vi "Treatment.vi"() -> ()   [LabVIEW 2020]
uses:
  controls/Rename.ctl
  controls/Load.ctl
  controls/CleanSD.ctl
  controls/Save.ctl
  controls/Del.ctl
  controls/Add.ctl
  controls/Average.ctl
  controls/mylistbox.ctl
  controls/SliderSDII.ctl
  controls/Calc.ctl
  controls/AllOffOn.ctl
  controls/Scale_up.ctl
  controls/Norm.ctl
  controls/LeftArrow.ctl
  controls/RightArrow.ctl
  Classes/Control/Control-Client/Control-Client.lvclass
  dependecies/ControlsVIs/Clusters-def/graphs_TR.ctl
  dependecies/ControlsVIs/Clusters-def/Graphs_ref_Client.ctl
  Classes/Control/Control-Client/Control-Client.lvclass/Control-Client.ctl
  Classes/Experiments/Experiments_group.lvclass/Experiments_group.ctl
  dependecies/ControlsVIs/Clusters-def/Types_of_Graphs-Client.ctl
  Classes/Control/Control-Client/methods/Read Group #.vi
  dependecies/globalVarSD.vi
  Classes/Control/Control-Client/Erase color.vi
  Classes/Experiments/Experiments_group.lvclass
panel:
  in  "stop":bool
  in  "VD2_calc_abs":bool
  in  "Right shift kinetics":T1
  in  "Left shift kinetics":T2
  in  "Norm Kinetics":T3
  in  "Scale_up":dbl=1.01 format="%#_3f"
  in  "ScaleUp":T4
  in  "Value":dbl=10.0 format="%#_13g"
  in  "ChangeAll":T5
  in  "NaN Correct":T6
  in  "CalcStability":T7
  out "stability":T8(graph)
  in  "X-scale":bool
  in  "Group title":string
  in  "Del group exp":T9
  in  "Add group":T10
  out "error out":errorcluster
  in  "Exp name":string
  in  "Clean mode":u16(ring)=1 items=["delete", "approx"]
  in  "Clean":T6
  in  "sigma":dbl=1.4 min=0.0 step=0.1
  in  "BG slider":T11={0.0, 16.0} scale=0.0..10.0
  in  "BG correct":T6
  in  "Del exp":T9
  in  "Load Exp":T12
  in  "Save exp":T13
  in  "Save":enum32{"Automatic", "User-def"}(ring)
  in  "Rename exp":T14
  in  "Average exp":T15
  in  "times slider":T11={120.7741935483871, 734.8387096774194} scale=-40.0..74.0 scale format="%#.1f"
  in  "del spec":i32=2 min=2 step=1
  in  "Del spectrum":T9
  in  "Add spectrum":T10
  out "Spectra":cluster{"Y":dbl[], "Y":dbl[]}[](graph)
  in  "waves slider":T11={434.19354838709677, 734.8387096774194} scale=240.824..813.9446 scale format="%#.1f"
  in  "del kin":i32=2 min=2 step=1
  in  "LogY":bool
  in  "Del kinetics":T9
  in  "Add kinetics":T10
  out "Kinetics":cluster{"Y":dbl[], "Y":dbl[]}[](graph)
  in  "folder of the day":string="no title"
  in  "selected wavelengths":dbl[](array[numeric])=[370.0, 400.0, 450.0, 500.0, 550.0, 600.0, 640.0, 700.0]
  out "Exp data graph":dbl[][](graph)
  in  "Commentaires exp":string="...Write experiment description..."
  in  "Experiments":T16=[4]
  in  "Group":u16(ring) items=["1. 17_05_2018-10-30-test"]
  in  "Tab Control":enum32{"Raw data"}(tab)
  in  "correct raw BG":bool
  out "Raw data":cluster{dbl[], dbl[]}[](graph)
  in  "raw bg":i32[](array[numeric])
  out "Raw data BG":cluster{dbl[], dbl[]}[](graph)
  # "copyrights: ELYSE Université Paris-Sud LCP/CNRS UMR8000 Dr. DENISOV Sergey"
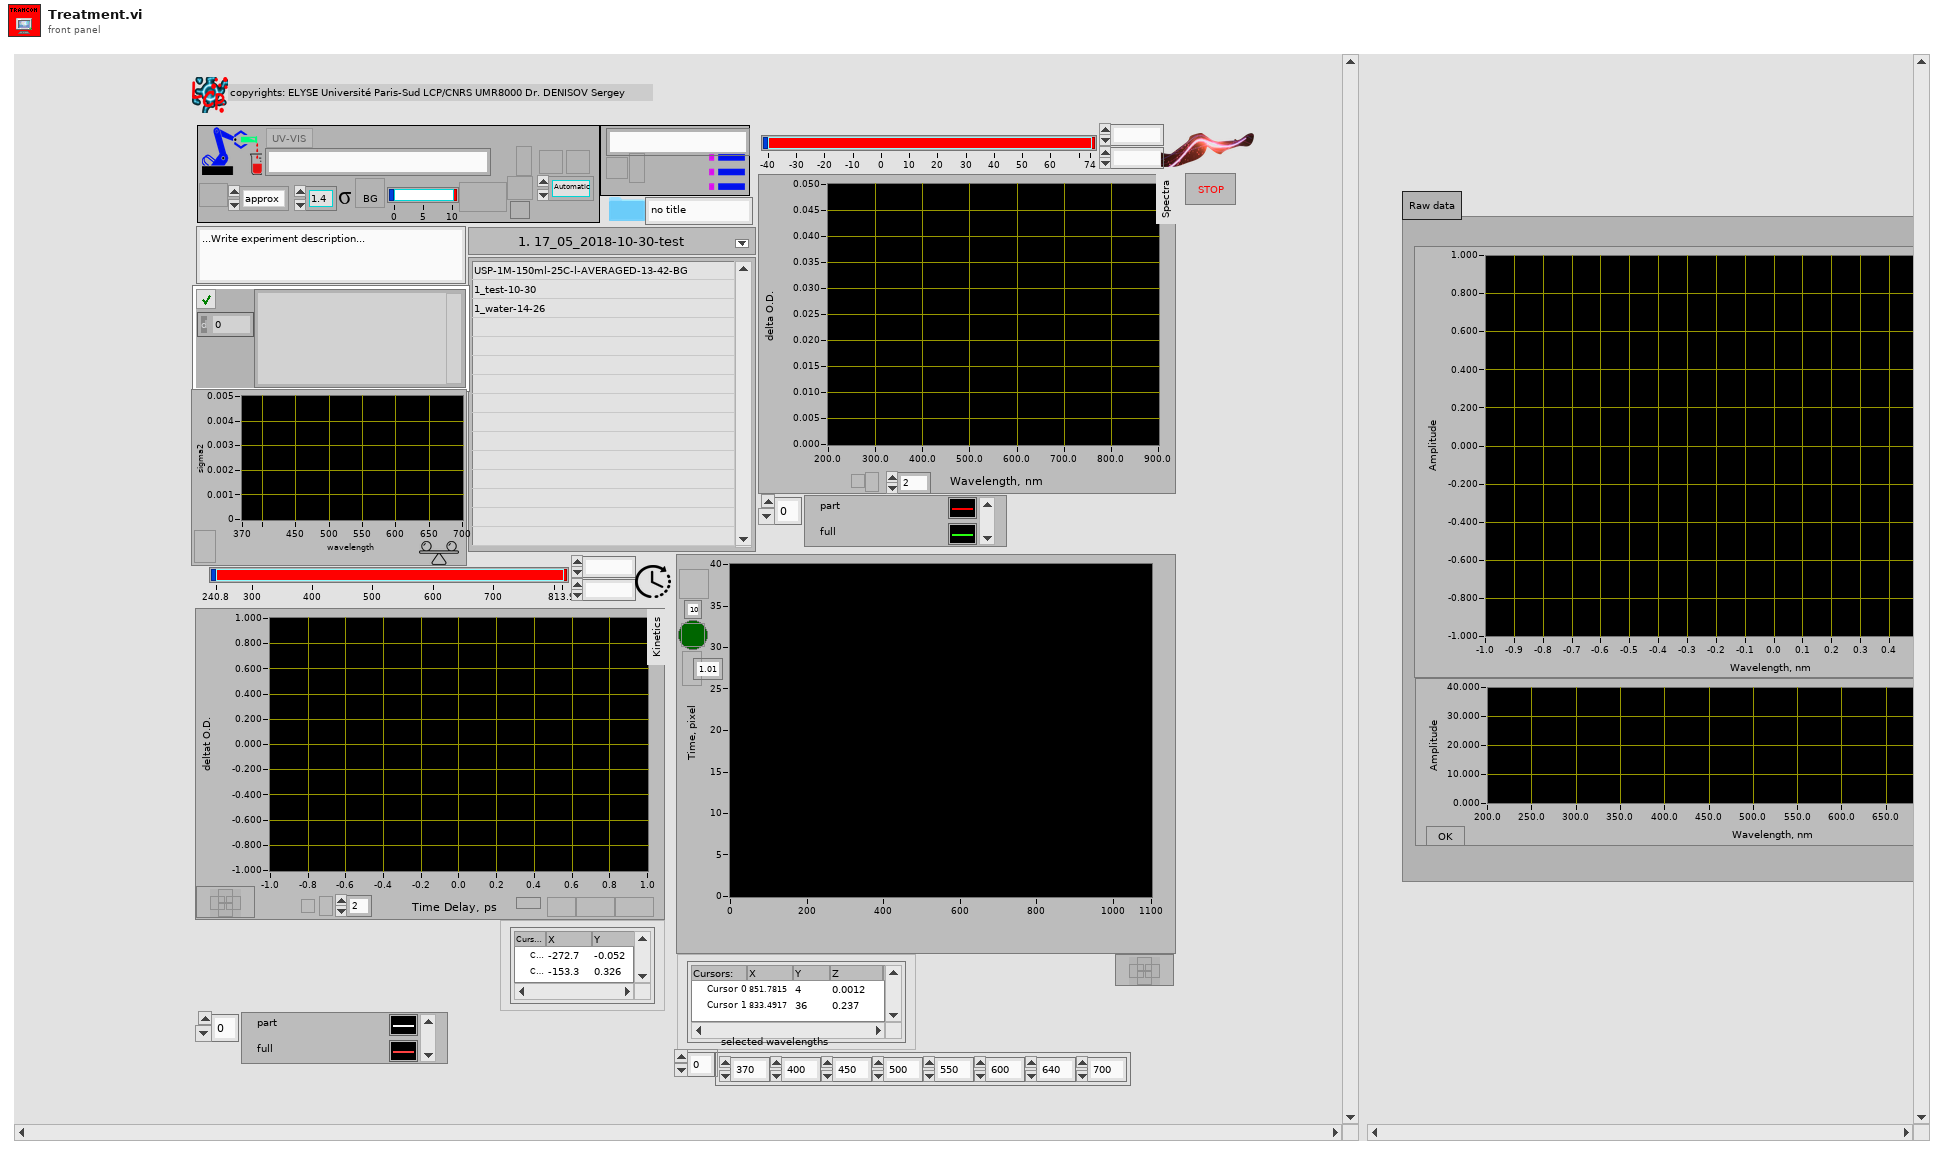
[diagram p1: front panel]
types:
  T1 = typedef "RightArrow.ctl" = bool
  T2 = typedef "LeftArrow.ctl" = bool
  T3 = typedef "Norm.ctl" = bool
  T4 = typedef "Scale_up.ctl" = bool
  T5 = typedef "AllOffOn.ctl" = bool
  T6 = typedef "CleanSD.ctl" = bool
  T7 = typedef "Calc.ctl" = bool
  T8 = cluster{"wavelengths":dbl[], "wavelengths":dbl[]}[]
  T9 = typedef "Del.ctl" = bool
  T10 = typedef "Add.ctl" = bool
  T11 = typedef "SliderSDII.ctl" = cluster{dbl, dbl}
  T12 = typedef "Load.ctl" = bool
  T13 = typedef "Save.ctl" = bool
  T14 = typedef "Rename.ctl" = bool
  T15 = typedef "Average.ctl" = bool
  T16 = typedef "mylistbox.ctl" = i32[]
  T17 = cluster{"waves slider":refnum<vi>, "times slider":refnum<vi>}
  T18 = typedef "Control-Client.lvclass/Graphs_ref_Client.ctl" = cluster{"Exp data graph ref":refnum<vi>, "Kinetics graph ref":refnum<vi>, "Spectrum graph ref":refnum<vi>, "cluster graph TR":T19, "Delays Graph":refnum<vi>, "Oscilloscope":refnum<vi>}
  T19 = typedef "graphs_TR.ctl" = cluster{"TR SC":refnum<vi>, "TR OD":refnum<vi>, "Raw data":refnum<vi>, "Raw data BG":refnum<vi>}
  T20 = cluster{"error out":refnum<vi>, "Experiments":refnum<vi>, "Group":refnum<vi>, "Commentaires exp":refnum<vi>}
  T21 = typedef "Control-Client.lvclass/Types_of_Graphs-Client.ctl" = string
  T22 = cluster{"Value":string, "Value":string, cluster{dbl, dbl, dbl, dbl}}
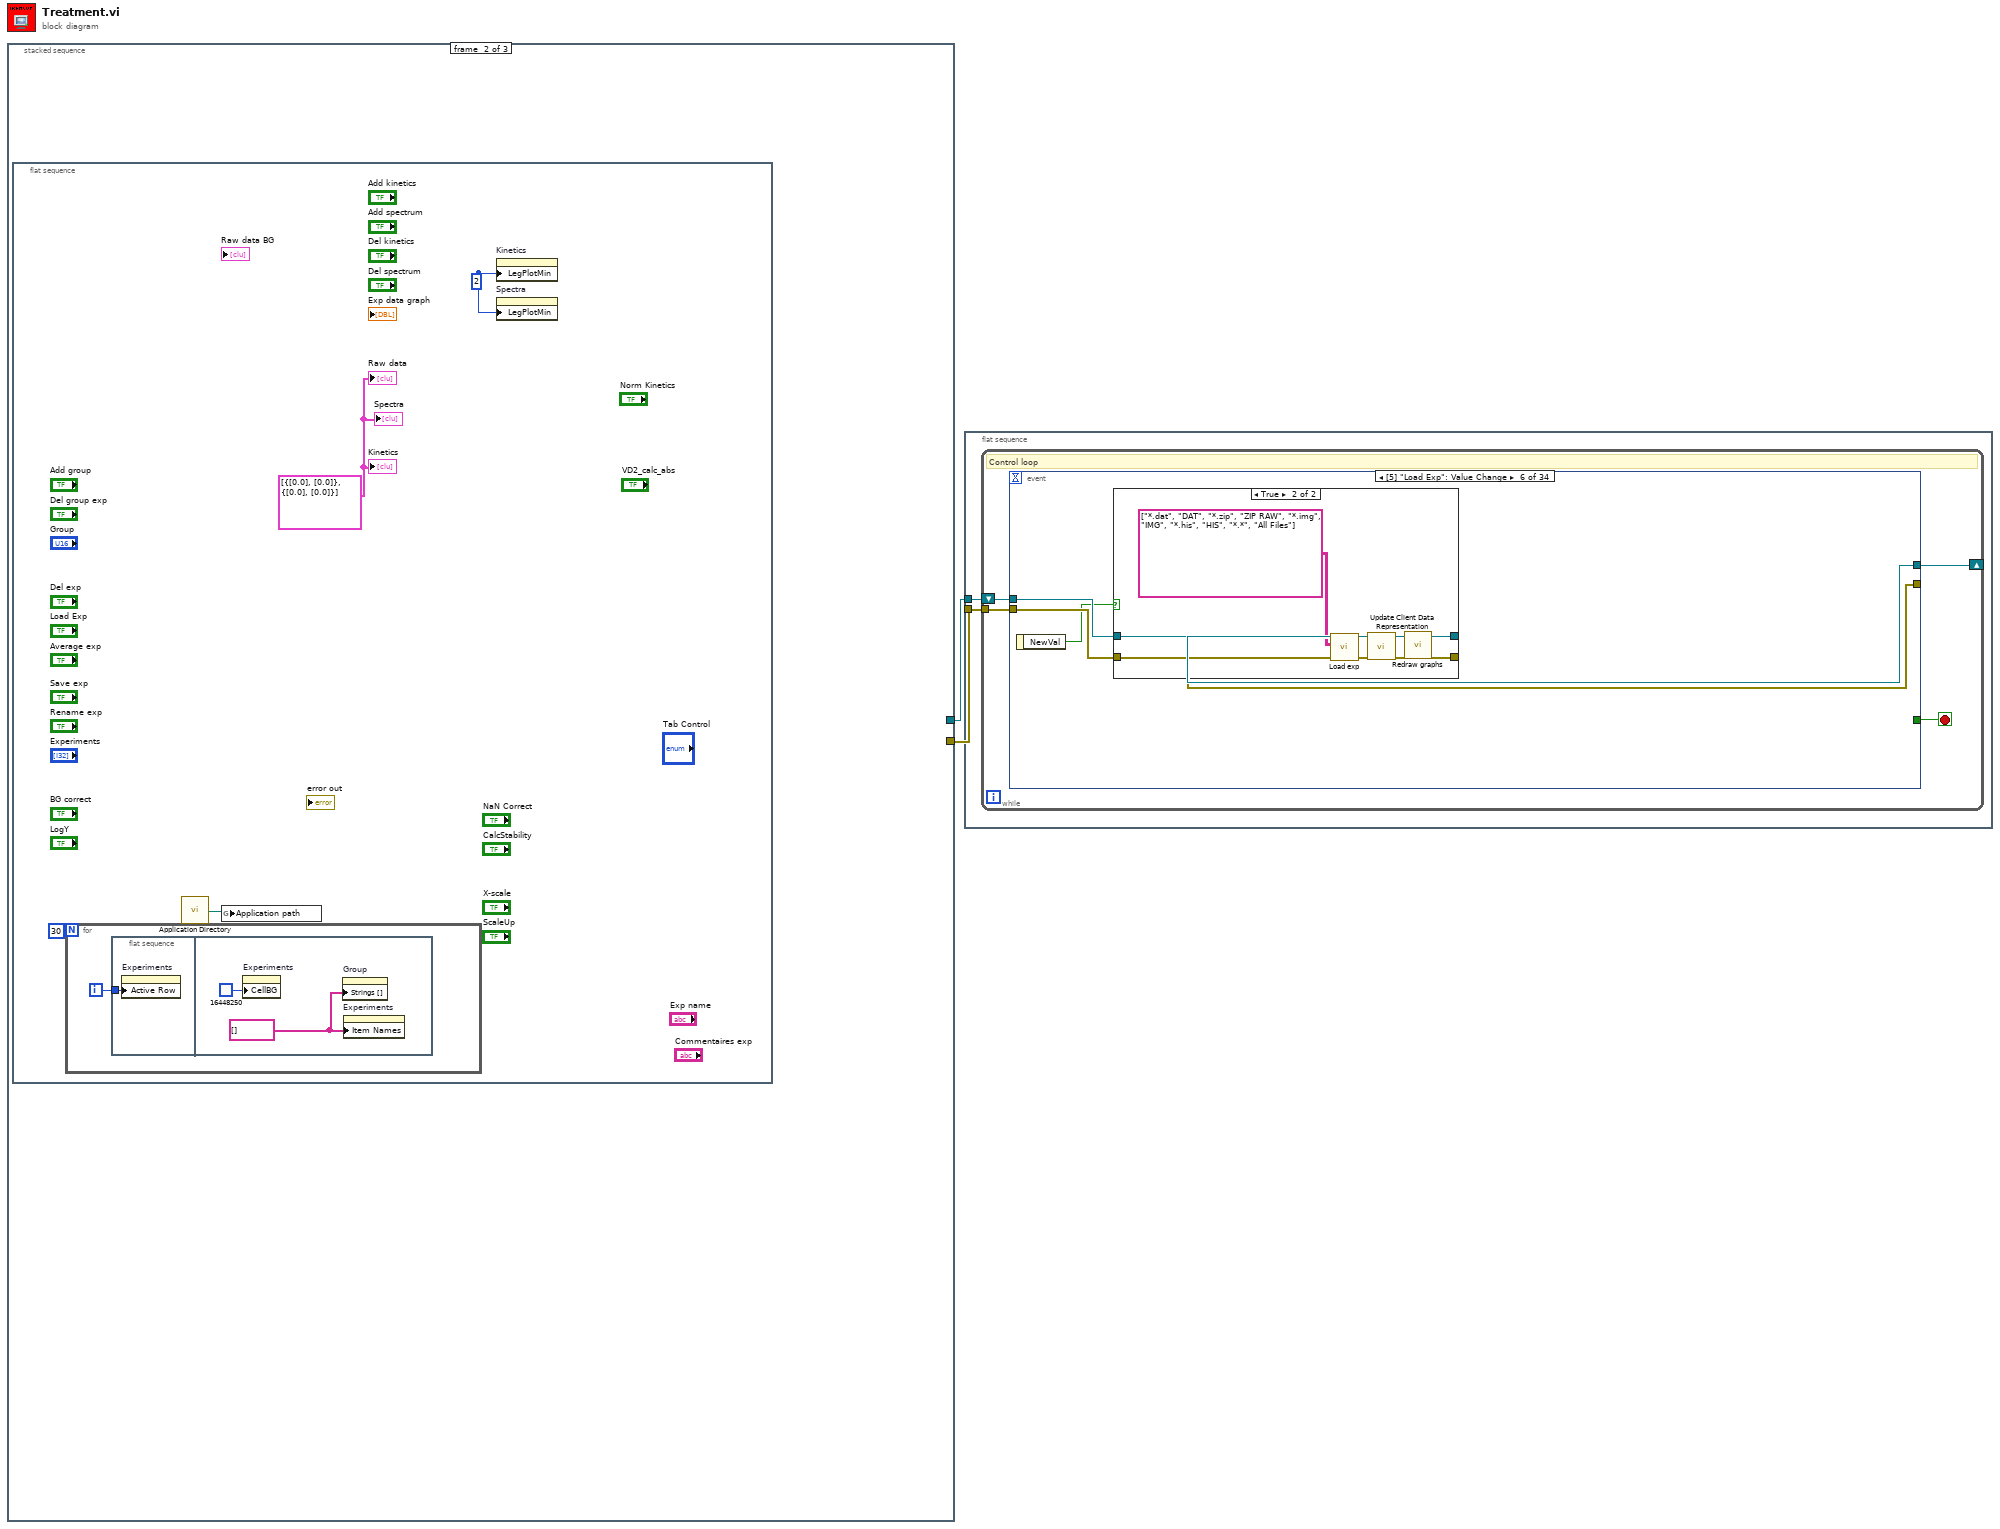
[diagram p0: block diagram]
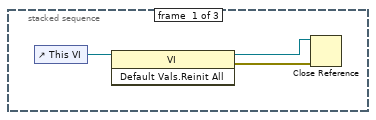
[diagram p2: hidden frame]
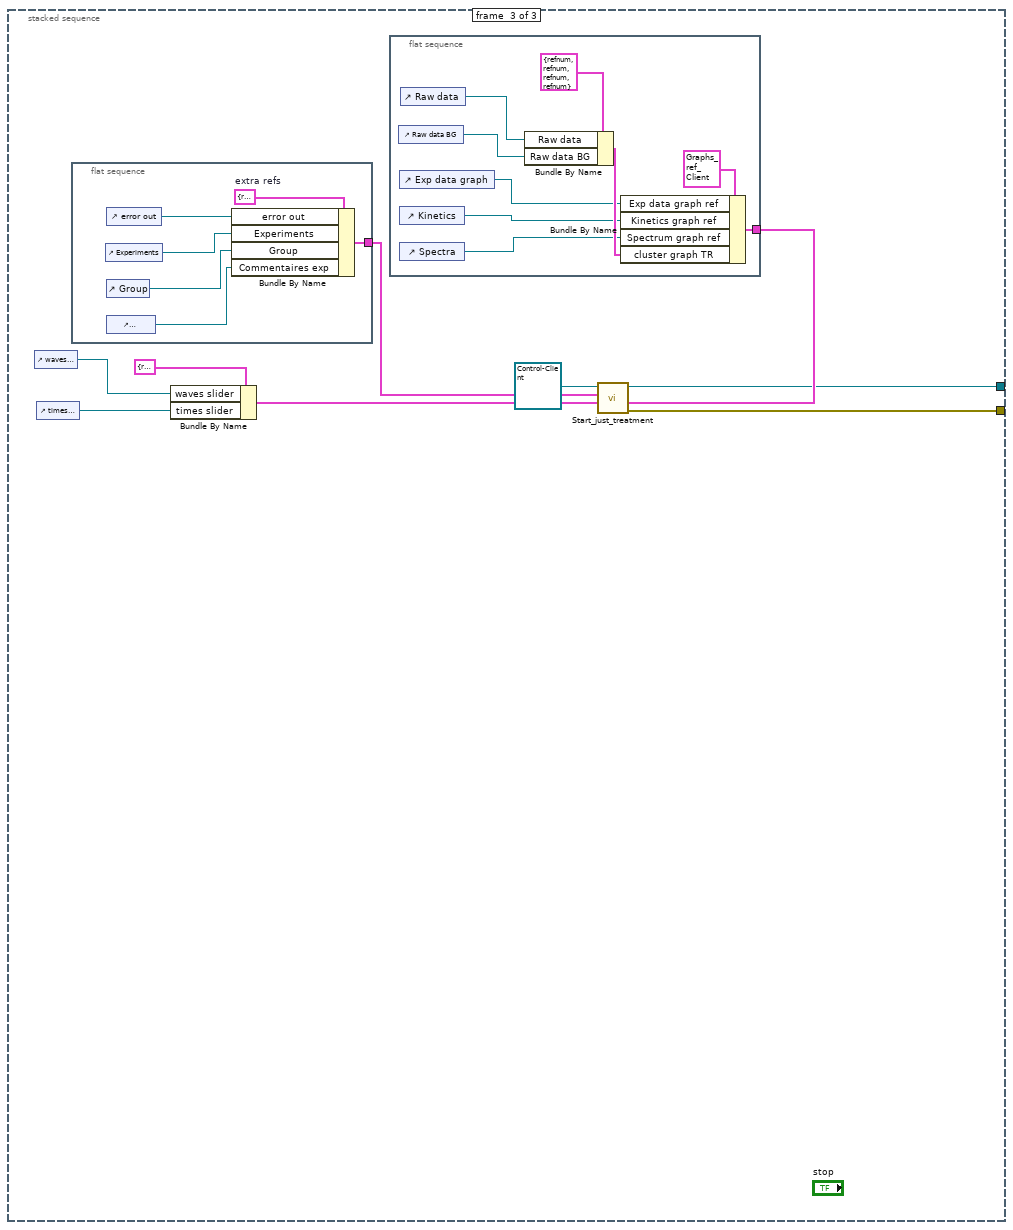
[diagram p3: hidden frame]
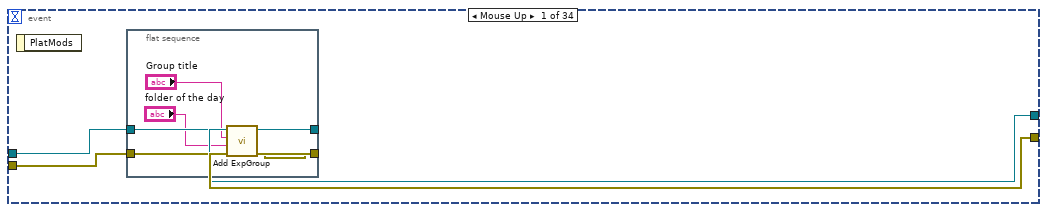
[diagram p4: hidden frame]
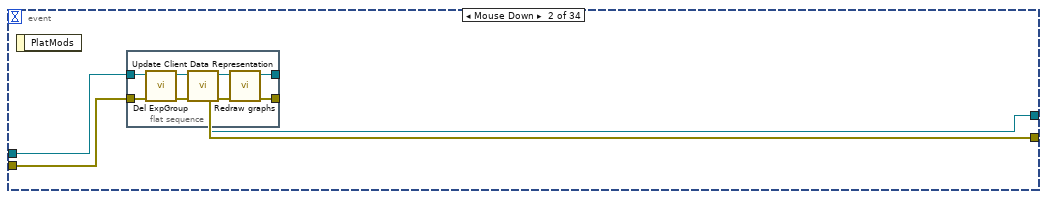
[diagram p5: hidden frame]
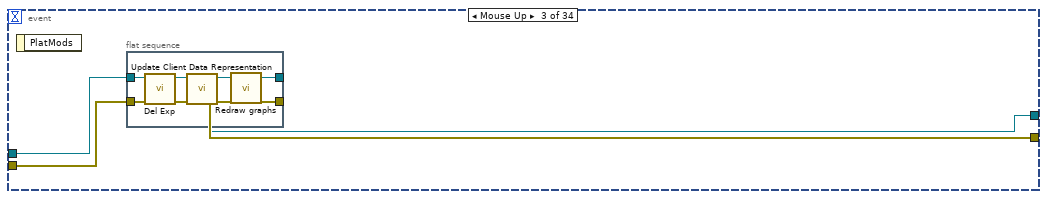
[diagram p6: hidden frame]
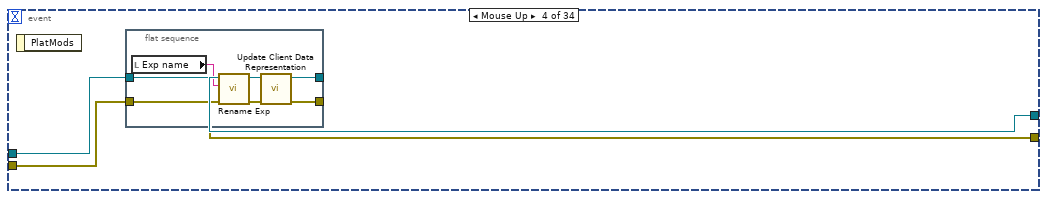
[diagram p7: hidden frame]
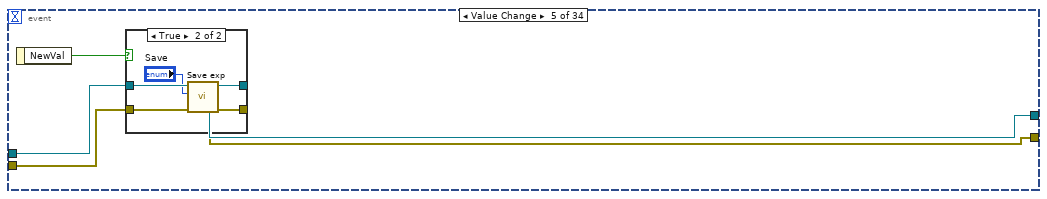
[diagram p8: hidden frame]
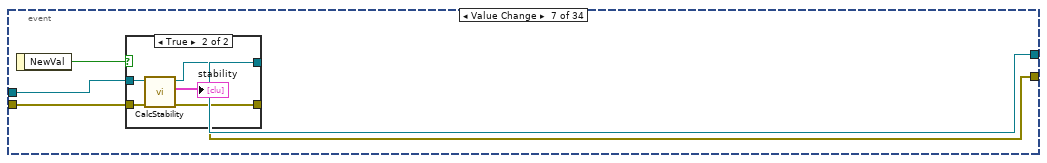
[diagram p11: hidden frame]
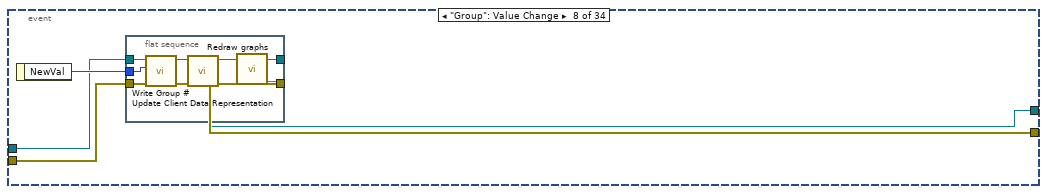
[diagram p13: hidden frame]
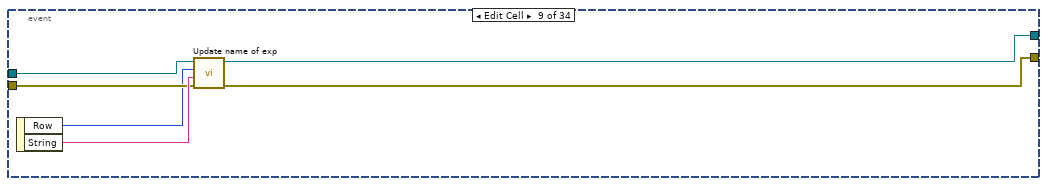
[diagram p14: hidden frame]
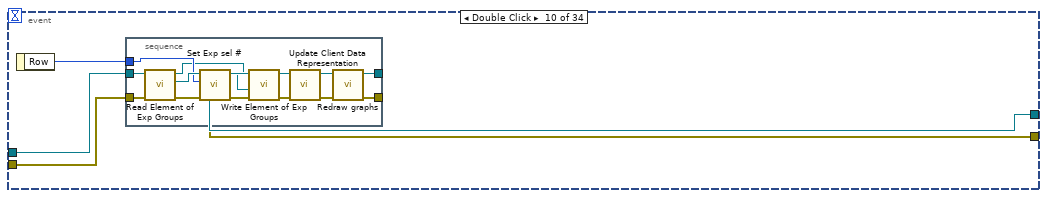
[diagram p15: hidden frame]
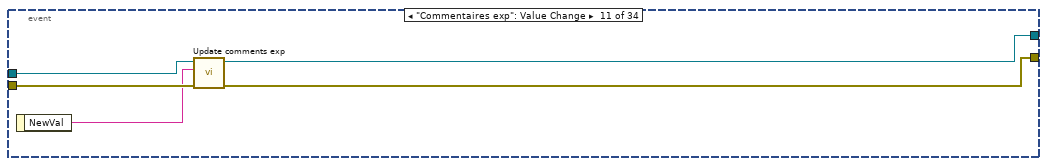
[diagram p16: hidden frame]
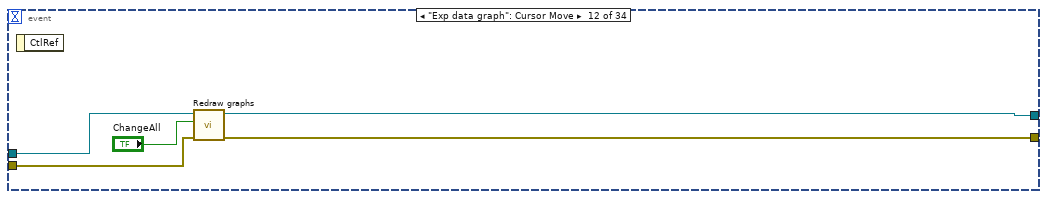
[diagram p17: hidden frame]
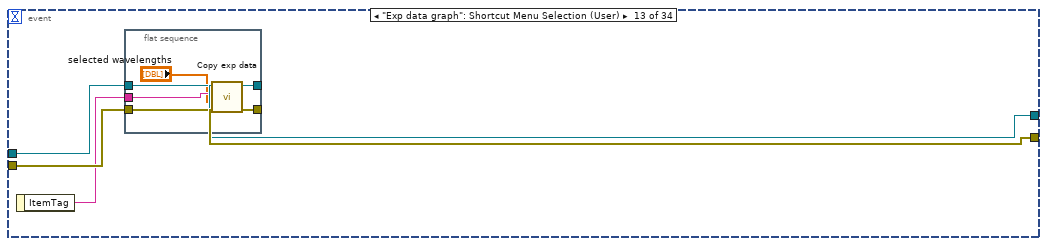
[diagram p18: hidden frame]
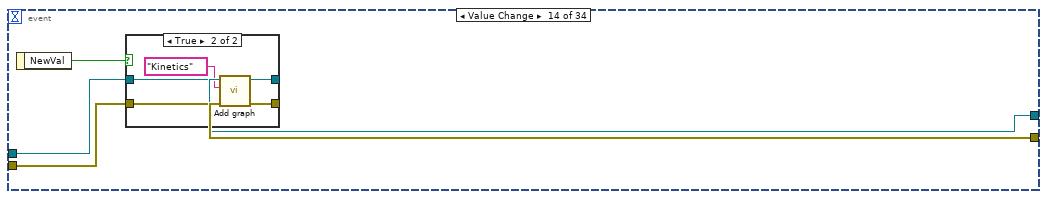
[diagram p19: hidden frame]
diagram:
  n1 = stacked-sequence {
    tunnel: [_ _ w14] -> w2
    tunnel: [_ _ w15] -> w1
    frame #0 {
      n2 = control-ref of="This VI"() -> (w5:refnum<vi>)
      n3 = invoke class="VI" method="Default Vals.Reinit All"(reference=w5) -> (reference out=w4:refnum<vi>, error out=w3:errorcluster)  [unwired: 2 in, 1 out]
      n4 = Close Reference(reference=w4, error in (no error)=w3) -> ()  [unwired: 1 out]
    }
    frame #1 {
      n5 = flat-sequence {
        frame #0 {
          w6 = cluster{dbl[], dbl[]}[] [{[0.0], [0.0]}, {[0.0], [0.0]}] ("Kinetics")
          w7 = u32 2 ("Legend:Plot Minimum")
          n6 = for {
            N: 30 -> [_]
            i -> [w10]
            n7 = flat-sequence {
              tunnel: w10 -> [w11]
              frame #0 {
                n8 = property on="Experiments" class="LstBox (strict)"("Active Row"=w11) -> ()  [unwired: 2 in, 2 out]
              }
              frame #1 {
                w12 = string[] [] ("Item Names")
                n9 = property on="Experiments" class="LstBox (strict)"("CellBG"=u32 16448250) -> ()  [unwired: 2 in, 2 out]
                n10 = property on="Group" class="Ring (strict)"("Strings []"=w12) -> ()  [unwired: 2 in, 2 out]
                n11 = property on="Experiments" class="LstBox (strict)"("Item Names"=w12) -> ()  [unwired: 2 in, 2 out]
              }
            }
          }
          n12 = call <vilib>:"Application Directory.vi"() -> ("Application Directory"=w9:path)
          n13 = global write "globalVarSD.vi" "Application path"(w9) -> ()
          n14 = property on="Kinetics" class="XYGraph (strict)"("LegPlotMin"=w7) -> ()  [unwired: 2 in, 2 out]
          n15 = property on="Spectra" class="XYGraph (strict)"("LegPlotMin"=w7) -> ()  [unwired: 2 in, 2 out]
          "Spectra" <- w6
          "Kinetics" <- w6
          "Raw data" <- w6
        }
      }
    }
    frame #2 {
      n16 = control-ref of="waves slider"() -> (w19:refnum<vi>)
      n17 = control-ref of="times slider"() -> (w20:refnum<vi>)
      n18 = flat-sequence {
        tunnel: [w23] -> w16
        frame #0 {
          w28 = T20 {"error out"=refnum, "Experiments"=refnum, "Group"=refnum, "Commentaires exp"=refnum}  # extra refs
          n19 = control-ref of="Experiments"() -> (w26:refnum<vi>)
          n20 = control-ref of="error out"() -> (w27:refnum<vi>)
          n21 = control-ref of="Group"() -> (w25:refnum<vi>)
          n22 = control-ref of="Commentaires exp"() -> (w24:refnum<vi>)
          n23 = Bundle By Name(cluster=w28, "error out"=w27, "Experiments"=w26, "Group"=w25, "Commentaires exp"=w24) -> (w23:T20)
        }
      }
      n24 = Bundle By Name(cluster=T17 {"waves slider"=refnum, "times slider"=refnum}, "waves slider"=w19, "times slider"=w20) -> (w18:T17)
      n25 = flat-sequence {
        tunnel: [w35] -> w17
        frame #0 {
          n26 = control-ref of="Raw data BG"() -> (w29:refnum<vi>)
          n27 = control-ref of="Exp data graph"() -> (w31:refnum<vi>)
          n28 = control-ref of="Kinetics"() -> (w33:refnum<vi>)
          n29 = control-ref of="Spectra"() -> (w32:refnum<vi>)
          n30 = control-ref of="Raw data"() -> (w30:refnum<vi>)
          n31 = Bundle By Name(cluster=T19 {"TR SC"=refnum, "TR OD"=refnum, "Raw data"=refnum, "Raw data BG"=refnum} ("cluster de sortie"), "Raw data"=w30, "Raw data BG"=w29) -> (w34:T19)
          n32 = Bundle By Name(cluster=T18 {"Exp data graph ref"=refnum, "Kinetics graph ref"=refnum, "Spectrum graph ref"=refnum, "cluster graph TR"={"TR SC"=refnum, "TR OD"=refnum, "Raw data"=refnum, "Raw data BG"=refnum}, "Delays Graph"=refnum, "Oscilloscope"=refnum} ("Graph refs"), "Exp data graph ref"=w31, "Kinetics graph ref"=w33, "Spectrum graph ref"=w32, "cluster graph TR"=w34) -> (w35:T18)
        }
      }
      n33 = call "Start_just_treatment.vi"("Graph refs"=w17, "Slider cluster"=w18, "extra refs"=w16, "Control-Client in"=refnum<class "Control-Client.lvclass"> refnum) -> ("error out"=w14:errorcluster, "Control-Client out"=w15:refnum<class "Control-Client.lvclass">)  [unwired: 6 in]
    }
  }
  n34 = flat-sequence {
    tunnel: w2 -> [w39]
    tunnel: w1 -> [w38]
    frame #0 {
      n35 = while "Control Loop" {
        tunnel: w39 -> [w43]
        shift-right: [w41] -> _
        shift-left: w38 -> [w42]
        stop <- w40 stop-if-true
        # "Control loop"
        n36 = event shown="[5] \"Load Exp\": Value Change" {
          selector: _ -> [_ _ _ _ _ _ _ _ _ _ _ _ _ _ _ _ _ _ _ _ _ _ _ _ _ _ _ _ _ _ _ _ _ _]
          dyn-events: _ -> [_ _ _ _ _ _ _ _ _ _ _ _ _ _ _ _ _ _ _ _ _ _ _ _ _ _ _ _ _ _ _ _ _ _]
          timeout: _ -> [_ _ _ _ _ _ _ _ _ _ _ _ _ _ _ _ _ _ _ _ _ _ _ _ _ _ _ _ _ _ _ _ _ _]
          tunnel: w43 -> [w47 w57 w67 w80 w89 w104 w117 w129 w146 w152 w171 w176 w181 w191 w203 w213 w230 w263 w276 w288 w298 w301 w307 w317 w341 w371 w383 w412 w428 w439 w447 w460 w494 w504]
          tunnel: [w46 w55 w69 w78 w90 w102 w118 w132 w145 w149 w170 w173 w180 w190 w202 w214 w226 w261 w274 w287 w298 w301 w306 w316 w339 w372 w384 w413 w427 w439 w445 w459 w495 w504] -> _
          tunnel: w42 -> [w45 w56 w66 w81 w92 w105 w120 w130 w147 w151 w172 w177 w182 w192 w204 w216 w228 w264 w277 w289 w299 w302 w308 w318 w342 w374 w386 w415 w429 w440 w448 w461 w492 w505]
          tunnel: [w44 w54 w68 w79 w91 w103 w119 w131 w144 w150 w169 w175 w178 w189 w201 w215 w227 w262 w275 w290 w299 w302 w305 w315 w340 w373 w385 w414 w426 w440 w446 w462 w493 w505] -> w41
          tunnel: [_ _ _ _ _ _ _ _ _ _ _ _ _ _ _ _ _ _ _ _ _ _ _ _ _ _ _ _ _ _ _ _ _ w503] -> w40
          event Mouse Up {
            n37 = event-data() -> ()  [unwired: 1 in, 1 out]
            n38 = flat-sequence {
              tunnel: w47 -> [w53]
              tunnel: [w49] -> w46
              tunnel: w45 -> [w52]
              tunnel: [w50] -> w44
              frame #0 {
                n39 = call "Add ExpGroup.vi"("error in (no error)"=w53, "folder of the day"="folder of the day", "Group title"="Group title", "Control-Client in"=w52) -> ("error out"=w49:errorcluster, "Control-Client out"=w50:refnum<class "Control-Client.lvclass">)  [unwired: 6 in]
              }
            }
          }
          event Mouse Down {
            n40 = event-data() -> ()  [unwired: 1 in, 1 out]
            n41 = flat-sequence {
              tunnel: w57 -> [w65]
              tunnel: w56 -> [w64]
              tunnel: [w63] -> w55
              tunnel: [w62] -> w54
              frame #0 {
                n42 = call "Del ExpGroup.vi"("error in (no error)"=w65, "Control-Client in"=w64) -> ("error out"=w58:errorcluster, "Control-Client out"=w59:refnum<class "Control-Client.lvclass">)  [unwired: 8 in]
                n43 = call "Update Client Data Representation.vi"("error in (no error)"=w58, "Control-Client in"=w59) -> ("error out"=w61:errorcluster, "Control-Client out"=w60:refnum<class "Control-Client.lvclass">)  [unwired: 8 in]
                n44 = call "Redraw graphs.vi"("error in (no error)"=w61, "Control-Client in"=w60) -> ("error out"=w63:errorcluster, "Control-Client out"=w62:refnum<class "Control-Client.lvclass">)  [unwired: 8 in]
              }
            }
          }
          event Mouse Up {
            n45 = event-data() -> ()  [unwired: 1 in, 1 out]
            n46 = flat-sequence {
              tunnel: [w77] -> w69
              tunnel: [w76] -> w68
              tunnel: w67 -> [w75]
              tunnel: w66 -> [w74]
              frame #0 {
                n47 = call "Del Exp.vi"("error in (no error)"=w75, "Control-Client in"=w74) -> ("error out"=w72:errorcluster, "Control-Client out"=w73:refnum<class "Control-Client.lvclass">)  [unwired: 8 in]
                n48 = call "Update Client Data Representation.vi"("error in (no error)"=w72, "Control-Client in"=w73) -> ("error out"=w71:errorcluster, "Control-Client out"=w70:refnum<class "Control-Client.lvclass">)  [unwired: 8 in]
                n49 = call "Redraw graphs.vi"("error in (no error)"=w71, "Control-Client in"=w70) -> ("error out"=w77:errorcluster, "Control-Client out"=w76:refnum<class "Control-Client.lvclass">)  [unwired: 8 in]
              }
            }
          }
          event Mouse Up {
            n50 = event-data() -> ()  [unwired: 1 in, 1 out]
            n51 = flat-sequence {
              tunnel: w81 -> [w88]
              tunnel: w80 -> [w87]
              tunnel: [w86] -> w79
              tunnel: [w85] -> w78
              frame #0 {
                n52 = local read "Exp name"() -> (w84:string)
                n53 = call "Rename Exp.vi"("error in (no error)"=w87, "New exp name"=w84, "Control-Client in"=w88) -> ("error out"=w82:errorcluster, "Control-Client out"=w83:refnum<class "Control-Client.lvclass">)  [unwired: 7 in]
                n54 = call "Update Client Data Representation.vi"("error in (no error)"=w82, "Control-Client in"=w83) -> ("error out"=w85:errorcluster, "Control-Client out"=w86:refnum<class "Control-Client.lvclass">)  [unwired: 8 in]
              }
            }
          }
          event Value Change {
            n55 = event-data() -> ("NewVal"=w93:T13)  [unwired: 1 in]
            n56 = case shown="True" w93 {
              tunnel: w92 -> [w95 w100]
              tunnel: [w95 w99] -> w91
              tunnel: [w94 w96] -> w90
              tunnel: w89 -> [w94 w98]
              frame False {
              }
              frame True {
                n57 = call "Save exp.vi"("error in (no error)"=w98, "save"="Save", "Control-Client in"=w100) -> ("error out"=w96:errorcluster, "Control-Client out"=w99:refnum<class "Control-Client.lvclass">)  [unwired: 7 in]
              }
            }
          }
          event Value Change {
            n58 = event-data() -> ("NewVal"=w101:T12)  [unwired: 1 in]
            n59 = case shown="True" w101 {
              tunnel: w105 -> [w107 w116]
              tunnel: w104 -> [w106 w115]
              tunnel: [w107 w109] -> w103
              tunnel: [w106 w110] -> w102
              frame False {
              }
              frame True {
                n60 = call "Load exp.vi"("error in (no error)"=w115, "Files of Type"=string[][] [["*.dat", "DAT"], ["*.zip", "ZIP RAW"], ["*.img", "IMG"], ["*.his", "HIS"], ["*.*", "All Files"]], "Control-Client in"=w116) -> ("error out"=w112:errorcluster, "Control-Client out"=w113:refnum<class "Control-Client.lvclass">)  [unwired: 7 in]
                n61 = call "Update Client Data Representation.vi"("error in (no error)"=w112, "Control-Client in"=w113) -> ("error out"=w111:errorcluster, "Control-Client out"=w114:refnum<class "Control-Client.lvclass">)  [unwired: 8 in]
                n62 = call "Redraw graphs.vi"("error in (no error)"=w111, "Control-Client in"=w114) -> ("error out"=w110:errorcluster, "Control-Client out"=w109:refnum<class "Control-Client.lvclass">)  [unwired: 8 in]
              }
            }
          }
          event Value Change {
            n63 = event-data() -> ("NewVal"=w121:T7)  [unwired: 1 in]
            n64 = case shown="True" w121 {
              tunnel: [w123 w126] -> w119
              tunnel: w120 -> [w123 w125]
              tunnel: [w122 w127] -> w118
              tunnel: w117 -> [w122 w128]
              frame False {
              }
              frame True {
                n65 = call "CalcStability.vi"("error in (no error)"=w128, "Control-Client in"=w125) -> ("error out"=w127:errorcluster, "stability"=→"stability":T8, "Control-Client out"=w126:refnum<class "Control-Client.lvclass">)  [unwired: 7 in]
              }
            }
          }
          event "Group": Value Change {
            n66 = event-data() -> ("NewVal"=w133:u16)  [unwired: 1 in]
            n67 = flat-sequence {
              tunnel: w133 -> [w138]
              tunnel: [w134] -> w132
              tunnel: [w135] -> w131
              tunnel: w130 -> [w140]
              tunnel: w129 -> [w139]
              frame #0 {
                n68 = call "Write Group #.vi"("error in (no error)"=w139, "Group #"=w138, "Control-Client in"=w140) -> ("error out"=w142:errorcluster, "Control-Client out"=w141:refnum<class "Control-Client.lvclass">)  [unwired: 7 in]
                n69 = call "Update Client Data Representation.vi"("error in (no error)"=w142, "Control-Client in"=w141) -> ("error out"=w137:errorcluster, "Control-Client out"=w136:refnum<class "Control-Client.lvclass">)  [unwired: 8 in]
                n70 = call "Redraw graphs.vi"("error in (no error)"=w137, "Control-Client in"=w136) -> ("error out"=w134:errorcluster, "Control-Client out"=w135:refnum<class "Control-Client.lvclass">)  [unwired: 8 in]
              }
            }
          }
          event Edit Cell {
            n71 = event-data() -> ("Row"=w143:i32, "String"=w148:string)  [unwired: 1 in]
            n72 = call "Update name of exp.vi"("error in (no error)"=w146, "Exp name"=w148, "Exp #"=w143, "Control-Client in"=w147) -> ("error out"=w145:errorcluster, "Control-Client out"=w144:refnum<class "Control-Client.lvclass">)  [unwired: 6 in]
          }
          event Double Click {
            n73 = event-data() -> ("Row"=w153:i32)  [unwired: 1 in]
            n74 = stacked-sequence {
              tunnel: w153 -> [w166]
              tunnel: w152 -> [w164]
              tunnel: w151 -> [w163]
              tunnel: [w154] -> w150
              tunnel: [w155] -> w149
              frame #0 {
                n75 = call "Read Element of Exp Groups.vi"("error in (no error)"=w164, "Control-Client in"=w163) -> ("error out"=w165:errorcluster, "Experiments_group.lvclass"=w167:refnum<class "Experiments_group.lvclass">, "Control-Client out"=w161:refnum<class "Control-Client.lvclass">)  [unwired: 7 in]
                n76 = call "Set Exp sel #.vi"("error in (no error)"=w165, "Exp sel #"=w166, "Experiments_group in"=w167) -> ("error out"=w160:errorcluster, "Experiments_group out"=w162:refnum<class "Experiments_group.lvclass">)  [unwired: 7 in]
                n77 = call "Write Element of Exp Groups.vi"("error in (no error)"=w160, "Experiments_group.lvclass"=w162, "Control-Client in"=w161) -> ("error out"=w159:errorcluster, "Control-Client out"=w158:refnum<class "Control-Client.lvclass">)  [unwired: 7 in]
                n78 = call "Update Client Data Representation.vi"("error in (no error)"=w159, "Control-Client in"=w158) -> ("error out"=w156:errorcluster, "Control-Client out"=w157:refnum<class "Control-Client.lvclass">)  [unwired: 8 in]
                n79 = call "Redraw graphs.vi"("error in (no error)"=w156, "Control-Client in"=w157) -> ("error out"=w155:errorcluster, "Control-Client out"=w154:refnum<class "Control-Client.lvclass">)  [unwired: 8 in]
              }
            }
          }
          event "Commentaires exp": Value Change {
            n80 = event-data() -> ("NewVal"=w168:string)  [unwired: 1 in]
            n81 = call "Update comments exp.vi"("error in (no error)"=w171, "Commentaires"=w168, "Control-Client in"=w172) -> ("error out"=w170:errorcluster, "Control-Client out"=w169:refnum<class "Control-Client.lvclass">)  [unwired: 7 in]
          }
          event "Exp data graph": Cursor Move {
            n82 = event-data() -> ()  [unwired: 1 in, 1 out]
            n83 = call "Redraw graphs.vi"("error in (no error)"=w176, "ChangeAll"="ChangeAll", "Control-Client in"=w177) -> ("error out"=w173:errorcluster, "Control-Client out"=w175:refnum<class "Control-Client.lvclass">)  [unwired: 7 in]
          }
          event "Exp data graph": Shortcut Menu Selection (User) {
            n84 = event-data() -> ("ItemTag"=w179:string)  [unwired: 1 in]
            n85 = flat-sequence {
              tunnel: w182 -> [w188]
              tunnel: w181 -> [w187]
              tunnel: [w186] -> w180
              tunnel: [w185] -> w178
              tunnel: w179 -> [w184]
              frame #0 {
                n86 = call "Copy exp data.vi"("error in (no error)"=w187, "selected wavelengths"="selected wavelengths", "ItemTag"=w184, "Control-Client in"=w188) -> ("error out"=w186:errorcluster, "Control-Client out"=w185:refnum<class "Control-Client.lvclass">)  [unwired: 6 in]
              }
            }
          }
          event Value Change {
            n87 = event-data() -> ("NewVal"=w193:T10)  [unwired: 1 in]
            n88 = case shown="True" w193 {
              tunnel: w192 -> [w195 w200]
              tunnel: w191 -> [w194 w199]
              tunnel: [w194 w198] -> w190
              tunnel: [w195 w197] -> w189
              frame False {
              }
              frame True {
                n89 = call "Add graph.vi"("error in (no error)"=w199, "Combo Box"="Kinetics", "Control-Client in"=w200) -> ("error out"=w198:errorcluster, "Control-Client out"=w197:refnum<class "Control-Client.lvclass">)  [unwired: 7 in]
              }
            }
          }
          event Value Change {
            n90 = event-data() -> ("NewVal"=w205:T10)  [unwired: 1 in]
            n91 = case shown="True" w205 {
              tunnel: w204 -> [w207 w212]
              tunnel: w203 -> [w206 w211]
              tunnel: [w206 w210] -> w202
              tunnel: [w207 w209] -> w201
              frame False {
              }
              frame True {
                n92 = call "Add graph.vi"("error in (no error)"=w211, "Combo Box"="Spectra", "Control-Client in"=w212) -> ("error out"=w210:errorcluster, "Control-Client out"=w209:refnum<class "Control-Client.lvclass">)  [unwired: 7 in]
              }
            }
          }
          event Value Change {
            n93 = event-data() -> ("NewVal"=w217:T3)  [unwired: 1 in, 5 out]
            n94 = case shown="True" w217 {
              tunnel: w216 -> [w219 w225]
              tunnel: [w219 w224] -> w215
              tunnel: [w218 w223] -> w214
              tunnel: w213 -> [w218 w222]
              frame False {
              }
              frame True {
                n95 = local read "del kin"() -> (w220:i32)
                n96 = call "Norm graph.vi"("error in (no error)"=w222, "#kinetics"=w220, "Combo Box"="Kinetics", "Control-Client in"=w225) -> ("error out"=w223:errorcluster, "Control-Client out"=w224:refnum<class "Control-Client.lvclass">)  [unwired: 6 in]
              }
            }
          }
          event Value Change {
            n97 = event-data() -> ("CtlRef"=w231:refnum<vi>, "NewVal"=w229:variant)  [unwired: 1 in]
            n98 = flat-sequence {
              tunnel: w231 -> [w241]
              tunnel: w230 -> [w240]
              tunnel: w229 -> [w239]
              tunnel: w228 -> [w236]
              tunnel: [w235] -> w227
              tunnel: [w234] -> w226
              frame #0 {
                n99 = property class="Bool (strict)"(reference=w241, error in=w240) -> (error out=w238:errorcluster, "ClassName"=w232:string)  [unwired: 1 out]
                n100 = case shown="\"Boolean\"" w232 {
                  tunnel: [TRUE w256] -> w237
                  tunnel: [w254 w259] -> w233
                  tunnel: w239 -> [_ w258]
                  tunnel: w238 -> [w254 w257]
                  frame "Digital", Default {
                    (unwired) FALSE
                  }
                  frame "Boolean" {
                    n101 = Variant To Data(error in=w257, type=TRUE, Variant=w258) -> (data=w256:bool, error out=w259:errorcluster)
                  }
                }
                n102 = case shown="True" w237 {
                  tunnel: w236 -> [w243 w251]
                  tunnel: [w243 w250] -> w235
                  tunnel: [w242 w249] -> w234
                  tunnel: w233 -> [w242 w248]
                  frame False {
                  }
                  frame True {
                    n103 = case shown="False" "Left shift kinetics" {
                      tunnel: [0.5 -0.5] -> w244
                      frame False {
                      }
                      frame True {
                      }
                    }
                    n104 = local read "del kin"() -> (w247:i32)
                    n105 = call "Shift X kinetics.vi"("shift"=w244, "error in (no error)"=w248, "#kinetics"=w247, "Combo Box"="Kinetics", "Control-Client in"=w251) -> ("error out"=w249:errorcluster, "Control-Client out"=w250:refnum<class "Control-Client.lvclass">)  [unwired: 5 in]
                  }
                }
              }
            }
          }
          event Value Change {
            n106 = event-data() -> ("NewVal"=w265:T9)  [unwired: 1 in]
            n107 = case shown="True" w265 {
              tunnel: w264 -> [w267 w273]
              tunnel: w263 -> [w266 w272]
              tunnel: [w267 w270] -> w262
              tunnel: [w266 w269] -> w261
              frame False {
              }
              frame True {
                n108 = call "Del graph.vi"("error in (no error)"=w272, "selected graph"="del kin", "Combo Box"="Kinetics", "Control-Client in"=w273) -> ("error out"=w269:errorcluster, "Control-Client out"=w270:refnum<class "Control-Client.lvclass">)  [unwired: 6 in]
              }
            }
          }
          event Value Change {
            n109 = event-data() -> ("NewVal"=w278:T9)  [unwired: 1 in]
            n110 = case shown="True" w278 {
              tunnel: w277 -> [w280 w286]
              tunnel: w276 -> [w279 w285]
              tunnel: [w280 w283] -> w275
              tunnel: [w279 w282] -> w274
              frame False {
              }
              frame True {
                n111 = call "Del graph.vi"("error in (no error)"=w285, "selected graph"="del spec", "Combo Box"="Spectra", "Control-Client in"=w286) -> ("error out"=w282:errorcluster, "Control-Client out"=w283:refnum<class "Control-Client.lvclass">)  [unwired: 6 in]
              }
            }
          }
          event "Kinetics": Shortcut Menu Selection (User) {
            n112 = event-data() -> ("ItemTag"=w291:string)  [unwired: 1 in]
            n113 = flat-sequence {
              tunnel: w291 -> [w297]
              tunnel: [w295] -> w290
              tunnel: w289 -> [w294]
              tunnel: w288 -> [w293]
              tunnel: [w292] -> w287
              frame #0 {
                n114 = call "Copy from XY graph.vi"("error in (no error)"=w293, "ItemTag"=w297, "Type of graph"="Kinetics" ("Combo Box"), "Control-Client in"=w294) -> ("error out"=w292:errorcluster, "Control-Client out"=w295:refnum<class "Control-Client.lvclass">)  [unwired: 6 in]
              }
            }
          }
          event "Spectra": Plot Attribute Change {
            n115 = event-data() -> ("PlotIdx"=w300:i32)  [unwired: 1 in]
            n116 = property on="Spectra" class="XYGraph (strict)"("Active Plot"=w300) -> ()  [unwired: 2 in, 2 out]
          }
          event "Kinetics": Plot Attribute Change {
            n117 = event-data() -> ("PlotIdx"=w303:i32)  [unwired: 1 in]
            n118 = property on="Kinetics" class="XYGraph (strict)"("Active Plot"=w303) -> ()  [unwired: 2 in, 2 out]
          }
          event "Spectra": Shortcut Menu Selection (User) {
            n119 = event-data() -> ("ItemTag"=w304:string)  [unwired: 1 in]
            n120 = flat-sequence {
              tunnel: w308 -> [w314]
              tunnel: w307 -> [w313]
              tunnel: [w312] -> w306
              tunnel: [w311] -> w305
              tunnel: w304 -> [w310]
              frame #0 {
                n121 = call "Copy from XY graph.vi"("error in (no error)"=w313, "ItemTag"=w310, "Type of graph"=T21 "Spectra" ("Combo Box"), "Control-Client in"=w314) -> ("error out"=w312:errorcluster, "Control-Client out"=w311:refnum<class "Control-Client.lvclass">)  [unwired: 6 in]
              }
            }
          }
          event Value Change {
            n122 = event-data() -> ("NewVal"=w319:T15)  [unwired: 1 in]
            n123 = case shown="True" w319 {
              tunnel: [w321 w335] -> w315
              tunnel: w318 -> [w321 w336]
              tunnel: w317 -> [w320 w333]
              tunnel: [w320 w334] -> w316
              frame False {
              }
              frame True {
                n124 = local read "waves slider"() -> (w329:T11)
                n125 = local read "times slider"() -> (w326:T11)
                n126 = property on="Commentaires exp" class="Str"() -> ("Value"=w332:string)  [unwired: 2 in, 2 out]
                n127 = property on="Exp name" class="Str"() -> ("Value"=w331:string)  [unwired: 2 in, 2 out]
                n128 = Unbundle(w326) -> (w325:dbl, w324:dbl)
                n129 = Unbundle(w329) -> (w328:dbl, w327:dbl)
                n130 = Bundle "bounds"(w325, w324, w328, w327) -> (w323:cluster{dbl, dbl, dbl, dbl})  [unwired: 1 in]
                n131 = Bundle("Value"=w331, "Value"=w332, w323) -> (w322:T22)  [unwired: 1 in]
                n132 = call "Average experiments.vi"("error in (no error)"=w333, "sigma"="sigma", "Name+Comments+bounds"=w322, "Control-Client in"=w336) -> ("error out"=w334:errorcluster, "Control-Client out"=w335:refnum<class "Control-Client.lvclass">)  [unwired: 6 in]
              }
            }
          }
          event Value Change {
            n133 = event-data() -> ("CtlRef"=w338:refnum<vi>, "NewVal"=w337:variant)  [unwired: 1 in]
            n134 = flat-sequence {
              tunnel: w342 -> [w352]
              tunnel: w341 -> [w344]
              tunnel: [w348] -> w340
              tunnel: [w347] -> w339
              tunnel: w338 -> [w351]
              tunnel: w337 -> [w346]
              frame #0 {
                n135 = property class="Ctl"(reference=w351) -> ("ClassName"=w350:string)  [unwired: 1 in, 2 out]
                n136 = case shown="\"Boolean\"" w350 {
                  tunnel: [FALSE w369] -> w349
                  tunnel: w346 -> [_ w370]
                  tunnel: [TRUE w368] -> w345
                  tunnel: w344 -> [w363 w367]
                  tunnel: [w363 w366] -> w343
                  frame "Digital", Default {
                  }
                  frame "Boolean" {
                    w369 = TRUE
                    n137 = Variant To Data(error in=w367, type=w369, Variant=w370) -> (data=w368:bool, error out=w366:errorcluster)
                  }
                }
                n138 = case shown="True" w345 {
                  tunnel: w352 -> [w354 w362]
                  tunnel: w343 -> [w353 w361]
                  tunnel: w349 -> [_ w360]
                  tunnel: [w354 w359] -> w348
                  tunnel: [w353 w358] -> w347
                  frame False {
                  }
                  frame True {
                    n139 = Unbundle("BG slider") -> (w355:dbl, w356:dbl)
                    n140 = call "BG correction.vi"("Change?"=w360, "error in (no error)"=w361, "def pixel upper"=w356, "def pixel lower"=w355, "Control-Client in"=w362) -> ("error out"=w358:errorcluster, "Control-Client out"=w359:refnum<class "Control-Client.lvclass">)  [unwired: 5 in]
                  }
                }
              }
            }
          }
          event "correct raw BG": Value Change {
            n141 = event-data() -> ("NewVal"=w375:bool)  [unwired: 1 in, 2 out]
            n142 = case shown="True" w375 {
              tunnel: w374 -> [w377 w382]
              tunnel: [w377 w381] -> w373
              tunnel: [w376 w380] -> w372
              tunnel: w371 -> [w376 w379]
              frame False {
              }
              frame True {
                n143 = call "Raw_BG_correction.vi"("error in (no error)"=w379, "raw bg"="raw bg", "Control-Client in"=w382) -> ("error out"=w380:errorcluster, "Control-Client out"=w381:refnum<class "Control-Client.lvclass">)  [unwired: 7 in]
              }
            }
          }
          event Value Change; "Kinetics": Cursor Move {
            n144 = event-data() -> ("CtlRef"=w387:refnum<vi>)  [unwired: 1 in]
            n145 = flat-sequence {
              tunnel: w387 -> [w393]
              tunnel: w386 -> [w392]
              tunnel: [w391] -> w385
              tunnel: [w390] -> w384
              tunnel: w383 -> [w389]
              frame #0 {
                n146 = property class="Ctl"(reference=w393, error in=w389) -> (error out=w388:errorcluster, "ClassName"=w397:string)  [unwired: 1 out]
                n147 = case shown="\"XYGraph\", Default" w397 {
                  tunnel: [FALSE TRUE] -> w396
                  tunnel: [TRUE "Clean"] -> w395
                  tunnel: [w406 w409] -> w394
                  tunnel: w388 -> [w406 w409]
                  frame "XYGraph", Default {
                  }
                  frame "Boolean" {
                  }
                }
                n148 = case shown="True" w395 {
                  tunnel: w394 -> [w399 w404]
                  tunnel: w396 -> [_ w403]
                  tunnel: [w399 w400] -> w390
                  tunnel: w392 -> [w398 w405]
                  tunnel: [w398 w401] -> w391
                  frame False {
                  }
                  frame True {
                    n149 = call "CursorKinGraphMove.vi"("error in (no error)"=w404, "change"=w403, "Clean mode"="Clean mode", "Control-Client in"=w405) -> ("error out"=w400:errorcluster, "Control-Client out"=w401:refnum<class "Control-Client.lvclass">)  [unwired: 6 in]
                  }
                }
              }
            }
          }
          event Value Change {
            n150 = event-data() -> ()  [unwired: 1 in, 1 out]
            n151 = flat-sequence {
              tunnel: w415 -> [w424]
              tunnel: [w423] -> w414
              tunnel: [w422] -> w413
              tunnel: w412 -> [w421]
              frame #0 {
                n152 = local read "ChangeAll"() -> (w416:T5)
                n153 = Unbundle("waves slider") -> (w418:dbl, w417:dbl)
                n154 = call "Change FromToWave_or_Time.vi"("ChangeAll"=w416, "Combo Box"=T21 "Spectra", "error in (no error)"=w421, "To"=w417, "From"=w418, "Control-Client in"=w424) -> ("error out"=w422:errorcluster, "Control-Client out"=w423:refnum<class "Control-Client.lvclass">)  [unwired: 4 in]
              }
            }
          }
          event Value Change {
            n155 = event-data() -> ("NewVal"=w425:T11)  [unwired: 1 in]
            n156 = flat-sequence {
              tunnel: w429 -> [w438]
              tunnel: [w437] -> w426
              tunnel: [w436] -> w427
              tunnel: w428 -> [w435]
              tunnel: w425 -> [_]
              frame #0 {
                n157 = local read "ChangeAll"() -> (w430:T5)
                n158 = Unbundle("times slider") -> (w431:dbl, w432:dbl)
                n159 = call "Change FromToWave_or_Time.vi"("ChangeAll"=w430, "Combo Box"=T21 "Kinetics", "error in (no error)"=w435, "To"=w432, "From"=w431, "Control-Client in"=w438) -> ("error out"=w436:errorcluster, "Control-Client out"=w437:refnum<class "Control-Client.lvclass">)  [unwired: 4 in]
              }
            }
          }
          event "LogY": Value Change {
            n160 = event-data() -> ("NewVal"=w441:bool)  [unwired: 1 in]
            n161 = flat-sequence {
              tunnel: w441 -> [w443]
              frame #0 {
                n162 = Boolean To (0,1)(Boolean=w443) -> (0, 1=w442:i16)
                n163 = property on="Kinetics" class="XYGraph (strict)"("YScale.Mapping Mode"=w442) -> ()  [unwired: 2 in, 2 out]
              }
            }
          }
          event Value Change {
            n164 = event-data() -> ("NewVal"=w444:T6)  [unwired: 1 in]
            n165 = case shown="True" w444 {
              tunnel: w448 -> [w450 w456]
              tunnel: w447 -> [w449 w455]
              tunnel: [w450 w453] -> w446
              tunnel: [w449 w454] -> w445
              frame False {
              }
              frame True {
                n166 = local read "ChangeAll"() -> (w452:T5)
                n167 = call "NaNCorrect.vi"("error in (no error)"=w455, "Value"="Value", "CorrectAll"=w452, "Control-Client in"=w456) -> ("error out"=w454:errorcluster, "Control-Client out"=w453:refnum<class "Control-Client.lvclass">)  [unwired: 6 in]
              }
            }
          }
          event "Scale_up": Value Change {
            n168 = event-data() -> ("CtlRef"=w458:refnum<vi>, "NewVal"=w457:variant)  [unwired: 1 in]
            n169 = flat-sequence {
              tunnel: [w474] -> w462
              tunnel: w461 -> [w473]
              tunnel: w460 -> [w472]
              tunnel: [w471] -> w459
              tunnel: w458 -> [w470]
              tunnel: w457 -> [w469]
              frame #0 {
                n170 = property class="Ctl"(reference=w470, error in=w472) -> (error out=w463:errorcluster, "ClassName"=w468:string)  [unwired: 1 out]
                n171 = case shown="\"Boolean\"" w468 {
                  tunnel: [FALSE w490] -> w465
                  tunnel: [TRUE w486] -> w464
                  tunnel: [w483 w489] -> w466
                  tunnel: w469 -> [_ w488]
                  tunnel: w463 -> [w483 w487]
                  frame "Digital", Default {
                  }
                  frame "Boolean" {
                    w490 = TRUE
                    n172 = Variant To Data(error in=w487, type=w490, Variant=w488) -> (data=w486:bool, error out=w489:errorcluster)
                  }
                }
                n173 = case shown="True" w464 {
                  tunnel: w473 -> [w476 w482]
                  tunnel: w466 -> [w475 w481]
                  tunnel: [w475 w480] -> w471
                  tunnel: [w476 w479] -> w474
                  tunnel: "Scale_up" -> [_ w478]
                  tunnel: w465 -> [_ w477]
                  frame False {
                  }
                  frame True {
                    n174 = call "ScaleUp correction.vi"("error in (no error)"=w481, "Change?"=w477, "ScaleUp"=w478, "Control-Client in"=w482) -> ("error out"=w480:errorcluster, "Control-Client out"=w479:refnum<class "Control-Client.lvclass">)  [unwired: 6 in]
                  }
                }
              }
            }
          }
          event "VD2_calc_abs": Value Change {
            n175 = event-data() -> ("NewVal"=w491:bool)  [unwired: 1 in, 5 out]
            n176 = case shown="True" w491 {
              tunnel: [w497 w501] -> w495
              tunnel: w494 -> [w497 w502]
              tunnel: [w496 w499] -> w493
              tunnel: w492 -> [w496 w500]
              frame False {
              }
              frame True {
                n177 = property on="Exp name" class="Str"() -> ("Value"=w498:string)  [unwired: 2 in, 2 out]
                n178 = call "VD2_TRABS_Calc.vi"("error in (no error)"=w502, "Exp name"=w498, "Control-Client in"=w500) -> ("error out"=w501:errorcluster, "Control-Client out"=w499:refnum<class "Control-Client.lvclass">)  [unwired: 7 in]
              }
            }
          }
          event "stop": Value Change {
            n179 = event-data() -> ("NewVal"=w503:bool)  [unwired: 1 in, 5 out]
          }
        }
      }
    }
  }
